vi "LJUD U3RAW ReadDefaults.vi"(7 "Comm Settings":T1={"Open LabJack "=TRUE, "Address"="1", "FirstFound"=TRUE}, 8 "error in (no error)":errorcluster, 11 "Handle In":i32) -> (0 "error out":errorcluster, 3 "Handle Out":i32)   [LabVIEW 2020]
panel:
  in  "BlockNum (0-7)":i32 min=0 max=7 step=1
  out "Write Array":u8[](array[numeric]) format="%.0x"
  out "Read Array":u8[](array[numeric]) format="%.0x"
  # "Reads the power up defaults from flash. Refer to the ReadDefaults documentation for details the block numbers and the defaults data it returns. The U3 contains data in blocks 0-3.\n\nhttps://labjack.com/support/datasheets/u3/low-level-function-reference/readdefaults"
  # "Byte 6: Errorcode"
  # "Byte 8+: Data"
  # "If open is false,\nthen a valid\nhandle must be\npassed in."
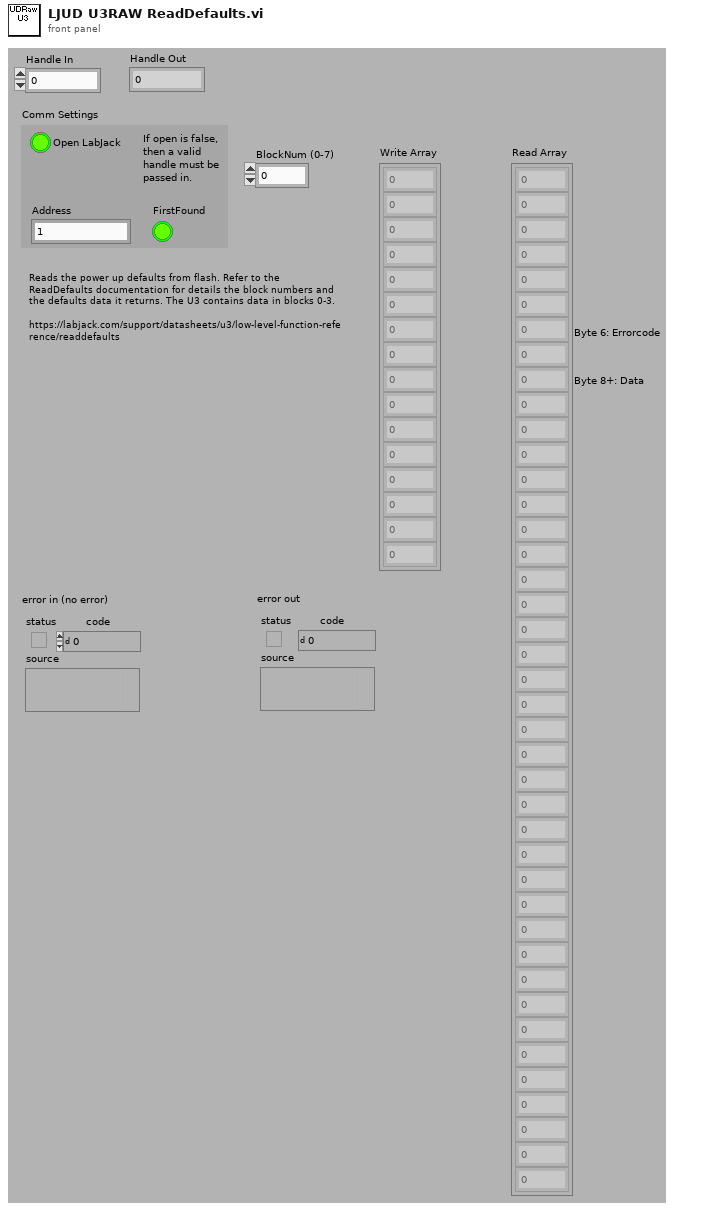
[diagram p1: front panel]
types:
  T1 = cluster{"Open LabJack ":bool, "Address":string, "FirstFound":bool}
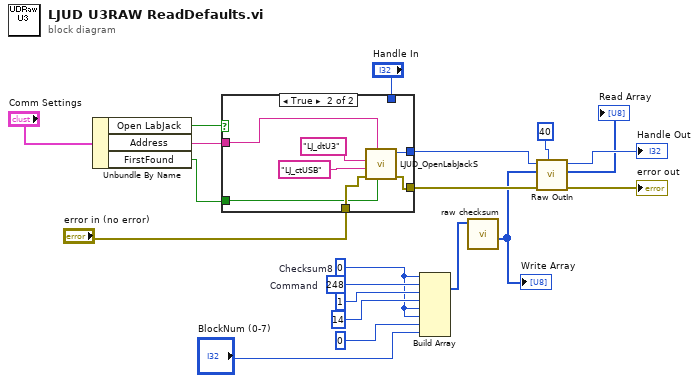
[diagram p0: block diagram]
diagram:
  w13 = u8 0  # Checksum8
  w20 = u8 248  # Command
  n1 = Unbundle By Name("Comm Settings") -> ("Open LabJack"=w11:bool, "Address"=w10:string, "FirstFound"=w9:bool)
  n2 = case shown="True" w11 {
    tunnel: w10 -> [_ w26]
    tunnel: "error in (no error)" -> [w22 w27]
    tunnel: [w22 w28] -> w7
    tunnel: [w21 w29] -> w6
    tunnel: w9 -> [_ w25]
    tunnel: "Handle In" -> [w21 _]
    frame False {
    }
    frame True {
      n3 = call "LJUD_OpenLabJackS.vi"("FirstFound"=w25, "Address"=w26, "error in"=w27, "ConnectionType"="LJ_ctUSB", "DeviceType"="LJ_dtU3") -> ("error out"=w28:errorcluster, "Handle"=w29:i32)  [unwired: 4 in, 1 out]
    }
  }
  n4 = Build Array(w13, w20, u8 1, u8 14, w13, w13, u8 0, "BlockNum (0-7)") -> (w16:i32[])
  n5 = call "raw checksum.vi"("Array"=w16) -> ("Array Output"=w2:u8[])  [unwired: 3 in, 7 out]
  "Write Array" <- w2
  n6 = call "Raw OutIn.vi"("# of bytes to read in"=40 ("# of bytes to read"), "error in"=w7, "Raw Out"=w2, "Handle In"=w6) -> ("error out"=→"error out":errorcluster, "Raw In"=→"Read Array":u8[], "Handle Out"=→"Handle Out":i32)  [unwired: 4 in, 1 out]
